vi "Get Status.vi"(8 "error in (no error)":errorcluster) -> (0 "error out":errorcluster, 1 "STATUS":u8, 2 "Encoder":i32)   [LabVIEW 2015, in "Tool Interface.lvlib"]
uses:
  Tool Interface.lvlib
  Tool Typedefs/_Motion STATUS Cluster--typedef.ctl
panel:
  out "Message":string
  # "STATUS Byte:\n0:  CRASH\n1:  NOPART\n2:  MOTION\n3:  FAULT\n4:  INSPECTSW\n5:  HOME\n6:  REV_LMT\n7:  FWD_LMT"
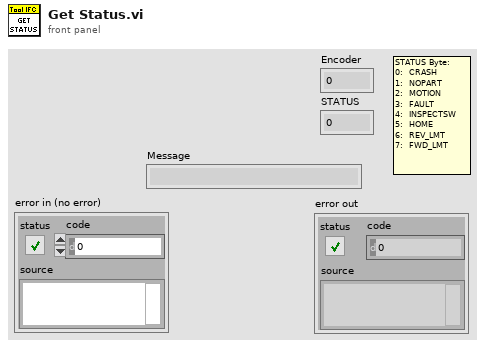
[diagram p1: front panel]
types:
  T1 = typedef "_Motion STATUS Cluster--typedef.ctl" = cluster{"Encoder":i32, "STATUS":u16, "MC SM State":u16, "M_Ctrl":u16}
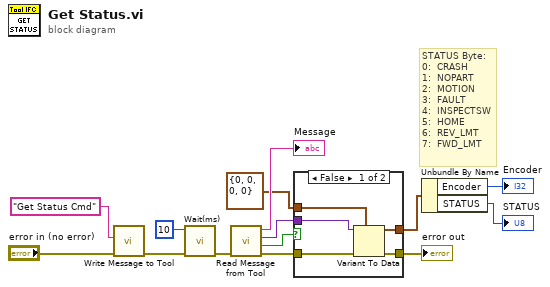
[diagram p0: block diagram]
diagram:
  # "STATUS Byte:\n0:  CRASH\n1:  NOPART\n2:  MOTION\n3:  FAULT\n4:  INSPECTSW\n5:  HOME\n6:  REV_LMT\n7:  FWD_LMT"
  n1 = call "Write Message to Tool.vi"("error in (no error)"="error in (no error)", "Message"="Get Status Cmd") -> ("error out"=w12:errorcluster)  [unwired: 9 in]
  n2 = call "Wait(ms).vi"("error in (no error)"=w12, "milliseconds"=u32 10) -> ("error out"=w11:errorcluster)  [unwired: 9 in]
  n3 = call "Read Message from Tool.vi"("error in (no error)"=w11) -> ("error out"=w8:errorcluster, "timed out?"=w6:bool, "Message Data"=w9:variant, "Message"=→"Message":string)  [unwired: 7 in]
  n4 = case shown="False" w6 {
    tunnel: w9 -> [w19 _]
    tunnel: w8 -> [w18 w20]
    tunnel: [w17 _] -> w3
    tunnel: [w16 w20] -> w7
    tunnel: T1 {"Encoder"=0, "STATUS"=0, "MC SM State"=0, "M_Ctrl"=0} ("_Motion Status Cluster--typedef") -> [w15 _]
    frame False {
      n5 = Variant To Data(error in=w18, type=w15, Variant=w19) -> (data=w17:T1, error out=w16:errorcluster)
    }
    frame True {
    }
  }
  "error out" <- w7
  n6 = Unbundle By Name(w3) -> ("Encoder"=→"Encoder":i32, "STATUS"=→"STATUS":u16)
